vi "Calculate_Area_Difference_Short_Subtracks(101-11)-1.vi"(4 "[IN] Areas particles\nPrimary Detected":dbl[][](array[numeric]), 5 "[IN] Start pos":i32, 6 "[IN] Primary \n(X,Y) Detected":dbl[][](array[numeric]), 7 "[IN] Subtrack":dbl[](array[numeric]), 8 "[IN] Index of \"101\" Dis-\nplacement in Subtrack":i32, 10 "[IN] Index of\n subtrack":i32, 11 "[IN] Areas \ndifference":dbl[](array[numeric])) -> (3 "[OUT] Areas differen\nce (101 + 11 points)":dbl[](array[numeric]))   [LabVIEW 2013]
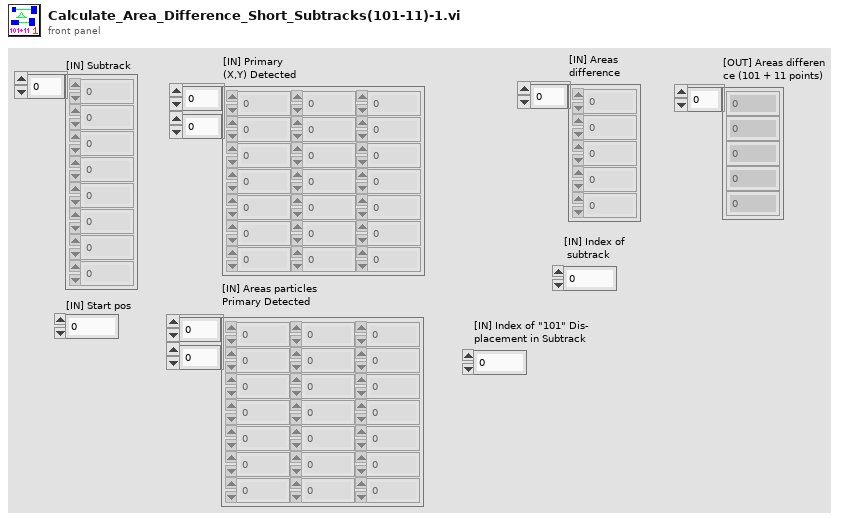
[diagram p1: front panel]
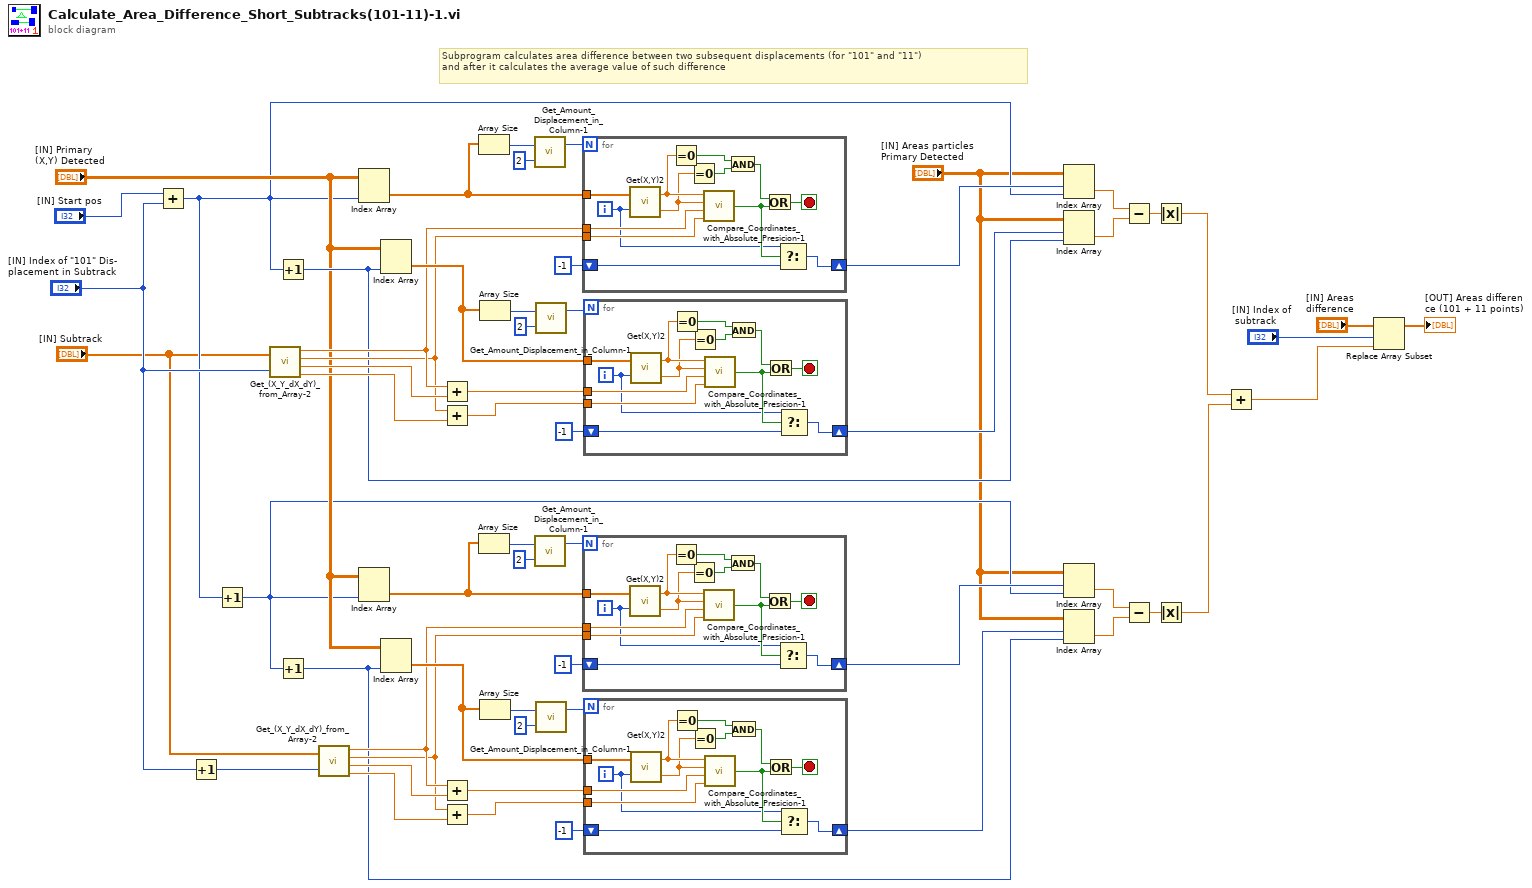
[diagram p0: block diagram]
diagram:
  # "Subprogram calculates area difference between two subsequent displacements (for \"101\" and \"11\") \nand after it calculates the average value of such difference"
  n1 = Add(x="[IN] Start pos", y="[IN] Index of \"101\" Dis-\nplacement in Subtrack") -> (x+y=w7:i32)
  n2 = Increment(x="[IN] Index of \"101\" Dis-\nplacement in Subtrack") -> (x+1=w8:i32)
  n3 = Increment(x=w7) -> (x+1=w6:i32)
  n4 = call "Get_(X_Y_dX_dY)_from_Array-2.vi"("(X,Y,dX,dY)"="[IN] Subtrack", "Index of Displacement"="[IN] Index of \"101\" Dis-\nplacement in Subtrack") -> ("X"=w39:dbl, "Y"=w35:dbl, "dX"=w38:dbl, "dY"=w34:dbl)
  n5 = Increment(x=w7) -> (x+1=w33:i32)
  n6 = Increment(x=w6) -> (x+1=w11:i32)
  n7 = call "Get_(X_Y_dX_dY)_from_Array-2.vi"("(X,Y,dX,dY)"="[IN] Subtrack", "Index of Displacement"=w8) -> ("X"=w17:dbl, "Y"=w13:dbl, "dX"=w16:dbl, "dY"=w12:dbl)
  n8 = Index Array(array="[IN] Primary \n(X,Y) Detected", index (col)=w7) -> (element=w54:dbl[])  [unwired: 1 in]
  n9 = Index Array(array="[IN] Primary \n(X,Y) Detected", index (col)=w6) -> (element=w28:dbl[])  [unwired: 1 in]
  n10 = Index Array(array="[IN] Primary \n(X,Y) Detected", index (col)=w33) -> (element=w48:dbl[])  [unwired: 1 in]
  n11 = Index Array(array="[IN] Primary \n(X,Y) Detected", index (col)=w11) -> (element=w23:dbl[])  [unwired: 1 in]
  n12 = Add(x=w39, y=w38) -> (x+y=w37:dbl)
  n13 = Add(x=w35, y=w34) -> (x+y=w36:dbl)
  n14 = Add(x=w17, y=w16) -> (x+y=w15:dbl)
  n15 = Add(x=w13, y=w12) -> (x+y=w14:dbl)
  n16 = Array Size(array=w54) -> (size(s)=w58:i32)
  n17 = Array Size(array=w28) -> (size(s)=w32:i32)
  n18 = Array Size(array=w48) -> (size(s)=w53:i32)
  n19 = Array Size(array=w23) -> (size(s)=w27:i32)
  n20 = call "Get_Amount_Displacement_in_Column-1.vi"("multiplier"=2, "# Rows"=w58) -> ("Displ amount"=w56:i32)  [unwired: 1 out]
  n21 = call "Get_Amount_Displacement_in_Column-1.vi"("multiplier"=2, "# Rows"=w32) -> ("Displ amount"=w30:i32)  [unwired: 1 out]
  n22 = call "Get_Amount_Displacement_in_Column-1.vi"("multiplier"=2, "# Rows"=w53) -> ("Displ amount"=w51:i32)  [unwired: 1 out]
  n23 = call "Get_Amount_Displacement_in_Column-1.vi"("multiplier"=2, "# Rows"=w27) -> ("Displ amount"=w25:i32)  [unwired: 1 out]
  n24 = for {
    N: w56 -> [_]
    tunnel: w54 -> [w70]
    tunnel: w39 -> [w69]
    tunnel: w35 -> [w68]
    shift-right: [w59] -> w47
    shift-left: -1 -> [w60]
    i -> [w61]
    stop <- w71 stop-if-true
    n25 = call "Get(X,Y)2.vi"("[IN] index of (X,Y)"=w61, "[IN] Array coordi\nnates (X,Y) in Frame"=w70) -> ("[OUT] Y"=w64:dbl, "[OUT] X"=w65:dbl)
    n26 = Equal To 0?(x=w65) -> (x = 0?=w67:bool)
    n27 = Equal To 0?(x=w64) -> (x = 0?=w66:bool)
    n28 = call "Compare_Coordinates_with_Absolute_Presicion-1.vi"("X 1"=w65, "Y 1"=w64, "X 2"=w69, "Y 2"=w68) -> ("[OUT] Same coordinates?"=w62:bool)  [unwired: 1 in]
    n29 = And(x=w67, y=w66) -> (x .and. y?=w63:bool)
    n30 = Or(x=w63, y=w62) -> (x .or. y?=w71:bool)
    n31 = Select(t=w61, s=w62, f=w60) -> (s? t:f=w59:i32)
  }
  n32 = for {
    N: w30 -> [_]
    tunnel: w28 -> [w83]
    tunnel: w17 -> [w82]
    tunnel: w13 -> [w81]
    shift-right: [w72] -> w22
    shift-left: -1 -> [w73]
    i -> [w74]
    stop <- w84 stop-if-true
    n33 = call "Get(X,Y)2.vi"("[IN] index of (X,Y)"=w74, "[IN] Array coordi\nnates (X,Y) in Frame"=w83) -> ("[OUT] Y"=w77:dbl, "[OUT] X"=w78:dbl)
    n34 = Equal To 0?(x=w78) -> (x = 0?=w80:bool)
    n35 = Equal To 0?(x=w77) -> (x = 0?=w79:bool)
    n36 = call "Compare_Coordinates_with_Absolute_Presicion-1.vi"("X 1"=w78, "Y 1"=w77, "X 2"=w82, "Y 2"=w81) -> ("[OUT] Same coordinates?"=w75:bool)  [unwired: 1 in]
    n37 = And(x=w80, y=w79) -> (x .and. y?=w76:bool)
    n38 = Or(x=w76, y=w75) -> (x .or. y?=w84:bool)
    n39 = Select(t=w74, s=w75, f=w73) -> (s? t:f=w72:i32)
  }
  n40 = for {
    N: w51 -> [_]
    tunnel: w48 -> [w96]
    tunnel: w37 -> [w95]
    tunnel: w36 -> [w94]
    shift-right: [w85] -> w46
    shift-left: -1 -> [w86]
    i -> [w87]
    stop <- w97 stop-if-true
    n41 = call "Get(X,Y)2.vi"("[IN] index of (X,Y)"=w87, "[IN] Array coordi\nnates (X,Y) in Frame"=w96) -> ("[OUT] Y"=w90:dbl, "[OUT] X"=w91:dbl)
    n42 = Equal To 0?(x=w91) -> (x = 0?=w93:bool)
    n43 = Equal To 0?(x=w90) -> (x = 0?=w92:bool)
    n44 = call "Compare_Coordinates_with_Absolute_Presicion-1.vi"("X 1"=w91, "Y 1"=w90, "X 2"=w95, "Y 2"=w94) -> ("[OUT] Same coordinates?"=w88:bool)  [unwired: 1 in]
    n45 = And(x=w93, y=w92) -> (x .and. y?=w89:bool)
    n46 = Or(x=w89, y=w88) -> (x .or. y?=w97:bool)
    n47 = Select(t=w87, s=w88, f=w86) -> (s? t:f=w85:i32)
  }
  n48 = for {
    N: w25 -> [_]
    tunnel: w23 -> [w109]
    tunnel: w15 -> [w108]
    tunnel: w14 -> [w107]
    shift-right: [w98] -> w21
    shift-left: -1 -> [w99]
    i -> [w100]
    stop <- w110 stop-if-true
    n49 = call "Get(X,Y)2.vi"("[IN] index of (X,Y)"=w100, "[IN] Array coordi\nnates (X,Y) in Frame"=w109) -> ("[OUT] Y"=w103:dbl, "[OUT] X"=w104:dbl)
    n50 = Equal To 0?(x=w104) -> (x = 0?=w106:bool)
    n51 = Equal To 0?(x=w103) -> (x = 0?=w105:bool)
    n52 = call "Compare_Coordinates_with_Absolute_Presicion-1.vi"("X 1"=w104, "Y 1"=w103, "X 2"=w108, "Y 2"=w107) -> ("[OUT] Same coordinates?"=w101:bool)  [unwired: 1 in]
    n53 = And(x=w106, y=w105) -> (x .and. y?=w102:bool)
    n54 = Or(x=w102, y=w101) -> (x .or. y?=w110:bool)
    n55 = Select(t=w100, s=w101, f=w99) -> (s? t:f=w98:i32)
  }
  n56 = Index Array(array="[IN] Areas particles\nPrimary Detected", index (row)=w47, index (col)=w7) -> (element=w45:dbl)
  n57 = Index Array(array="[IN] Areas particles\nPrimary Detected", index (row)=w46, index (col)=w33) -> (element=w44:dbl)
  n58 = Index Array(array="[IN] Areas particles\nPrimary Detected", index (row)=w22, index (col)=w6) -> (element=w20:dbl)
  n59 = Index Array(array="[IN] Areas particles\nPrimary Detected", index (row)=w21, index (col)=w11) -> (element=w19:dbl)
  n60 = Subtract(x=w45, y=w44) -> (x-y=w43:dbl)
  n61 = Subtract(x=w20, y=w19) -> (x-y=w18:dbl)
  n62 = Absolute Value(x=w43) -> (abs(x)=w5:dbl)
  n63 = Absolute Value(x=w18) -> (abs(x)=w4:dbl)
  n64 = Add(x=w5, y=w4) -> (x+y=w1:dbl)
  n65 = Replace Array Subset(array="[IN] Areas \ndifference", new element=w1, index="[IN] Index of\n subtrack") -> (→"[OUT] Areas differen\nce (101 + 11 points)":dbl[])
